vi "Fetch Measurement (Harmonics).vi"(6 "Timeout (10000 ms)":i32=10000 min=1, 8 "error in (no error)":errorcluster, 9 "Number of Item (1)":i32=1 min=1 max=32, 10 "Measure Item (1: Plural)":i32(ring)=1 items=["One", "Plural"], 11 "VISA resource name":refnum<visa-resource-name>) -> (0 "error out":errorcluster, 1 "Measurement":dbl[][](array[numeric]), 2 "Function":string[](array[string]), 3 "VISA resource name out":refnum<visa-resource-name>)   [LabVIEW 2023, in "Yokogawa WT300 Series.lvlib"]
doc: "Queries the harmonic measurement numeric list data.\n\n<B>Note:</B> This VI does not check the instrument status. If you want to check the instrument status, call the Error Query VI at the conclusion of the sequence."
uses:
  Yokogawa WT300 Series.lvlib
  Private/Measurement Data Convert (Harmonics).vi
panel:
  # "Total        DC            1             2              3             4"
  # "ms"
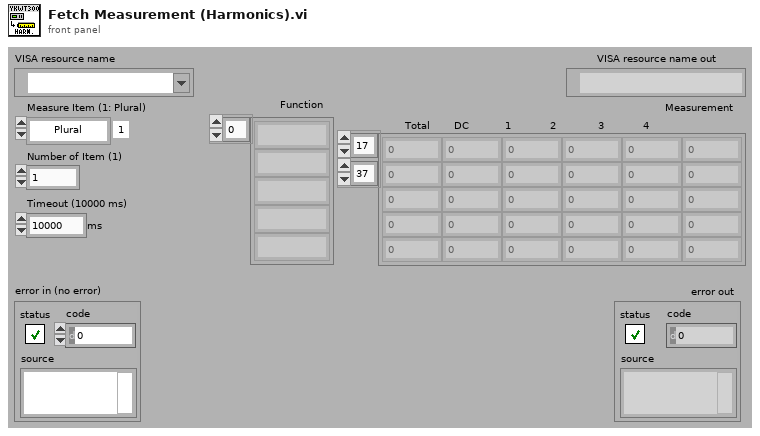
[diagram p1: front panel]
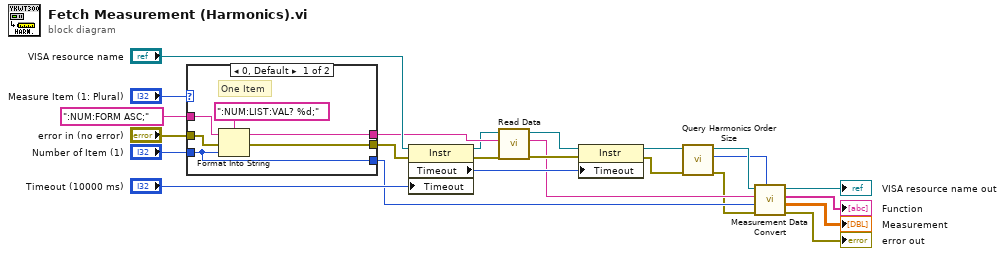
[diagram p0: block diagram]
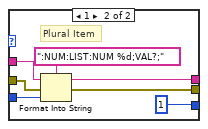
[diagram p2: hidden frame]
diagram:
  n1 = case shown="0, Default" "Measure Item (1: Plural)" {
    tunnel: ":NUM:FORM ASC;" ("形式文字列") -> [w29 w36]
    tunnel: "Number of Item (1)" -> [w25 w35]
    tunnel: "error in (no error)" -> [w28 w34]
    tunnel: [w27 w33] -> w14
    tunnel: [w26 w32] -> w19
    tunnel: [w25 1] -> w4
    frame 0, Default {
      # "One Item"
      n2 = Format Into String(format string=":NUM:LIST:VAL? %d;" ("形式文字列"), initial string=w29, error in=w28, w25) -> (resulting string=w27:string, error out=w26:errorcluster)
    }
    frame 1 {
      # "Plural Item"
      n3 = Format Into String(format string=":NUM:LIST:NUM %d;VAL?;" ("形式文字列"), initial string=w36, error in=w34, w35) -> (resulting string=w33:string, error out=w32:errorcluster)
    }
  }
  n4 = property on="プロパティノード" class="Instr"(reference="VISA resource name", error in=w19, "Timeout"="Timeout (10000 ms)") -> (reference out=w12:refnum<visa-resource-name>, error out=w13:errorcluster, "Timeout"=w18:u32)
  n5 = call "Read Data.vi"("error in (no error)"=w13, "Send Command (Empty)"=w14, "VISA resource name"=w12) -> ("error out"=w15:errorcluster, "Read Data"=w5:string, "VISA resource name out"=w16:refnum<visa-resource-name>)  [unwired: 5 in, 1 out]
  n6 = property on="プロパティノード" class="Instr"(reference=w16, error in=w15, "Timeout"=w18) -> (reference out=w11:refnum<visa-resource-name>, error out=w10:errorcluster)
  n7 = call "Query Harmonics Order Size.vi"("error in (no error)"=w10, "VISA resource name"=w11) -> ("error out"=w3:errorcluster, "Number of Harmonics Order"=w1:i32, "VISA resource name out"=w2:refnum<visa-resource-name>)  [unwired: 7 in]
  n8 = call-poly "Measurement Data Convert.vi"("Number of Harmonics Order (1)"=w1, "error in (no error)"=w3, "Item Number Offset (1)"=w4, "Measurement Data (Empty)"=w5, "VISA resource name"=w2) -> ("error out"=→"error out":errorcluster, "Measurement"=→"Measurement":dbl[][], "Function"=→"Function":string[], "VISA resource name out"=→"VISA resource name out":refnum<visa-resource-name>)  [unwired: 3 in]
